vi "To JPEG Stream.vi"(7 "Quality (85)":i32=85, 8 "error out":errorcluster, 11 "image data":T1) -> (0 "error out":errorcluster, 3 "data":string)   [LabVIEW 2020, in "LV Tiff.lvlib"]
uses:
  LV Tiff.lvlib
  <vilib>/picture/picture.llb/imagedata.ctl
  <vilib>/Dataflow_G/G-Image/G-Image.lvlib
  <vilib>/Dataflow_G/G-Image/Image IO/Polymorphic VIs/Save JPG Image (Memory).vi
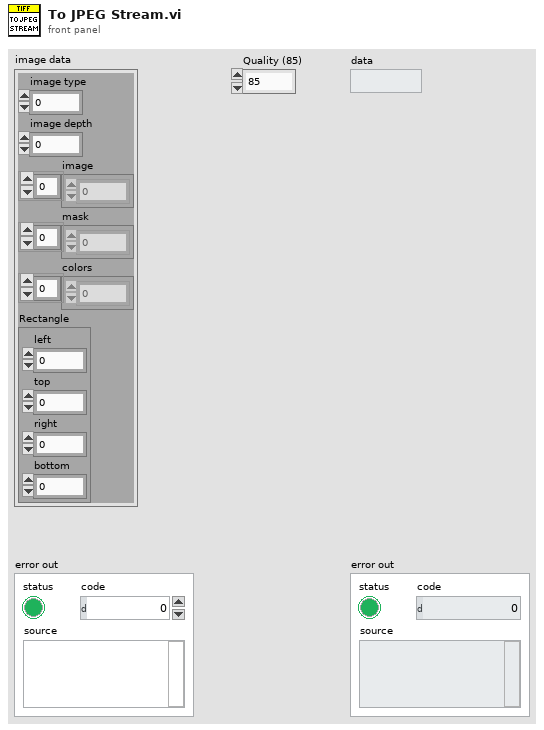
[diagram p1: front panel]
types:
  T1 = typedef "imagedata.ctl" = cluster{"image type":i32, "image depth":i32, "image":u8[], "mask":u8[], "colors":u32[], "Rectangle":cluster{"left":i16, "top":i16, "right":i16, "bottom":i16}}
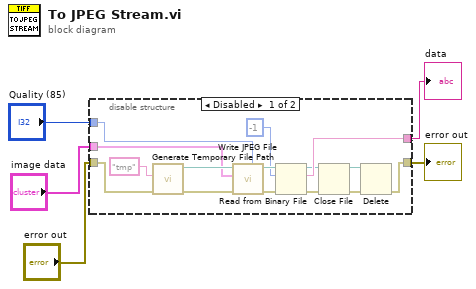
[diagram p0: block diagram]
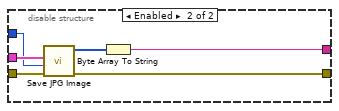
[diagram p2: hidden frame]
diagram:
  n1 = disable-structure shown="Disabled" {
    disable-tunnel: "image data" -> [w18 w26]
    disable-tunnel: [w13 w24] -> w4
    disable-tunnel: "error out" -> [w11 w23]
    disable-tunnel: [w10 w22] -> w2
    disable-tunnel: "Quality (85)" -> [w6 w21]
    frame Disabled {
      n2 = call <vilib>:"Generate Temporary File Path.vi"("error in (no error)"=w11, "Temporary File Extension (tmp)"="tmp") -> ("error out"=w17:errorcluster, "Unique Temporary File Path"=w19:path)  [unwired: 8 in]
      n3 = call <vilib>:"Write JPEG File.vi"("quality (80)"=w6, "error in (no error)"=w17, "image data"=w18, "path to JPEG file"=w19) -> ("error out"=w16:errorcluster, "path"=w15:path)  [unwired: 6 in]
      n4 = Read from Binary File(8:w16, 10:-1 ("count (1)"), 11:w15) -> (0:w12:errorcluster, 2:w13:string, 3:w8:refnum<file>)  [unwired: 3 in, 1 out]
      n5 = Close File(refnum=w8, error in=w12) -> (path=w7:path, error out=w9:errorcluster)
      n6 = Delete(path (use dialog)=w7, error in=w9) -> (error out=w10:errorcluster)  [unwired: 3 in, 2 out]
    }
    frame Enabled {
      n7 = call-poly <vilib>:"Save JPG Image.vi"("error in (no error)"=w23, "Quality (85)"=w21, "Image"=w26) -> ("error out"=w22:errorcluster, "Encoded Image"=w25:u8[])  [unwired: 7 in]
      n8 = Byte Array To String(unsigned byte array=w25) -> (string=w24:string)
    }
  }
  "data" <- w4
  "error out" <- w2
